vi "LVClass_ClosedLoopSecurity_SetData.vi"(0 "ClosedLoopSecurity in":refnum<class "ClosedLoopSecurity.lvclass">, 5 "ClosedLoopSecurityParams":T1, 11 "error in (no error)":errorcluster) -> (4 "ClosedLoopSecurity out":refnum<class "ClosedLoopSecurity.lvclass">, 15 "error out":errorcluster)   [LabVIEW 2020, in "ClosedLoopSecurity.lvclass"]
doc: "set tolerances\n\n<B>security_paramsIn</B> : Pointer to Closed Loop security params object.\n<B>security_paramsOut</B> : Pointer to Closed Loop security params object.\n<B>max_saturated_act_count</B> : Maximum tolerated count of saturated actuators\n<B>max_camera_fill_pct</B> : Maximum tolerated saturation percentage on camera signal\n<B>max_pupil_size_variation</B> : Maximum tolerated variation of the pupil size, relatively to the command\n matrix pupil size\n<B>max_dwf_pv</B> : Maximum tolerated delta wavefront peak-to-valley"
uses:
  ClosedLoopSecurity.lvclass
  Controls/ClosedLoopSecurityParameters.ctl
  ClosedLoopSecurity.lvclass/ClosedLoopSecurity.ctl
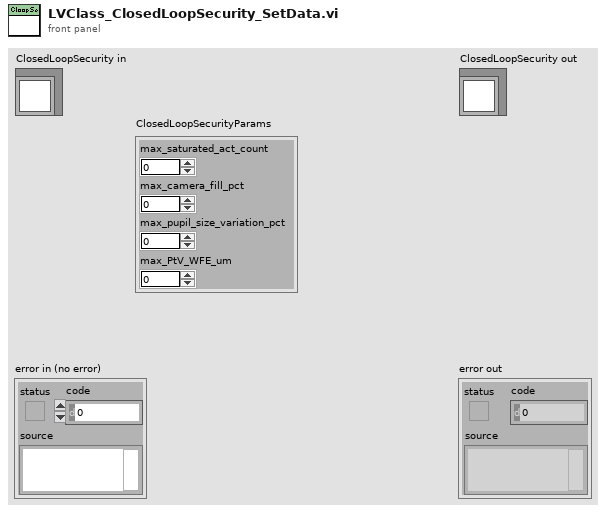
[diagram p1: front panel]
types:
  T1 = typedef "ClosedLoopSecurityParameters.ctl" = cluster{"max_saturated_act_count":i32, "max_camera_fill_pct":i32, "max_pupil_size_variation_pct":i32, "max_PtV_WFE_um":sgl}
  T2 = typedef "ClassID.ctl" = i64
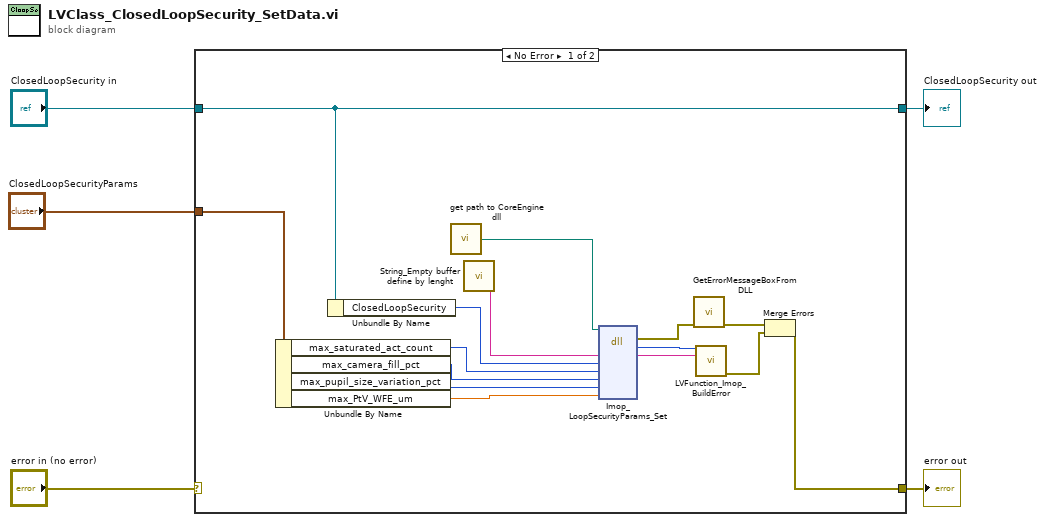
[diagram p0: block diagram]
diagram:
  n1 = case shown="No Error" "error in (no error)" {
    selector: "error in (no error)" -> [_ w22]
    tunnel: [w13 w22] -> w4
    tunnel: [w6 w21] -> w2
    tunnel: "ClosedLoopSecurity in" -> [w6 w21]
    tunnel: "ClosedLoopSecurityParams" -> [w12 _]
    frame No Error {
      n2 = Unbundle By Name(w12) -> ("max_saturated_act_count"=w11:i32, "max_camera_fill_pct"=w10:i32, "max_pupil_size_variation_pct"=w9:i32, "max_PtV_WFE_um"=w8:sgl)
      n3 = Unbundle By Name(w6) -> ("ClosedLoopSecurity"=w7:T2)
      n4 = call "get path to CoreEngine dll.vi"() -> ("path to wavekit library"=w14:path)  [unwired: 14 in, 1 out]
      n5 = call "String_Empty buffer define by lenght.vi"() -> ("Empty buffer"=w20:string)  [unwired: 1 in]
      n6 = dll-call lib="D:/soft/HASO_v3/SVN_trunk/ImOpCoreEngine4_LV2011/DLLs/c_interface_vc100.dll" fn="Imop_LoopSecurityParams_Set"(path in=w14, "message"=w20, "security_params"=w7, "max_saturated_act_count"=w11, "max_camera_fill_pct"=w10, "max_pupil_size_variation"=w9, "High_amplitude"=w8) -> (error out=w17:errorcluster, "return type"=w18:i32, "message"=w19:string)  [unwired: 7 in, 1 out]
      n7 = call "GetErrorMessageBoxFromDLL.vi"("error IN"=w17) -> ("error OUT"=w16:errorcluster)  [unwired: 10 in]
      n8 = call "LVFunction_Imop_BuildError.vi"("code"=w18, "String to Prepend to source (\"\")"=w19) -> ("error out"=w15:errorcluster)  [unwired: 13 in]
      n9 = Merge Errors(w16, w15) -> (w13:errorcluster)
    }
    frame Error {
    }
  }
  "error out" <- w4
  "ClosedLoopSecurity out" <- w2
